vi "Start.vi"(8 "error in (no error)":errorcluster, 10 "Message in":refnum<class "StartMessage.lvclass">, 11 "BMC in":refnum<class "BMC.lvclass">) -> (0 "error out":errorcluster, 3 "BMC out":refnum<class "BMC.lvclass">)   [LabVIEW 2012, in "BMC.lvclass"]
doc: "This member function is called when the statemachine in the run.vi receives an 'start' command. It relays the message to all observers of the component.\n\nOverride this member function in your derived class if you need additional start functionality (but don't forget to call the parent method)."
uses:
  BMC.lvclass
  <vilib>/Distrio/Murmex/StartMessage/StartMessage.lvclass
  <vilib>/Distrio/Murmex/Murmex/Murmex.lvclass
  BMC.lvclass/BMC.ctl
panel:
  # "This member function is called when the statemachine in the run.vi receives an 'start' command. It relays the message to all observers of the component.\n\nOverride this member function in your derived class if you need additional start functionality (but don't forget to call the parent method)."
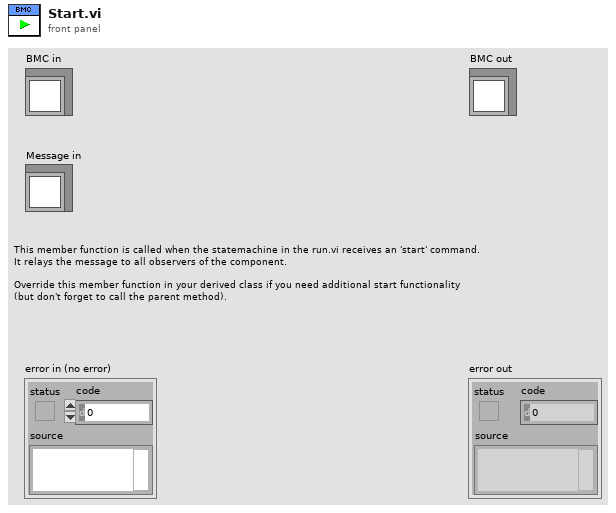
[diagram p1: front panel]
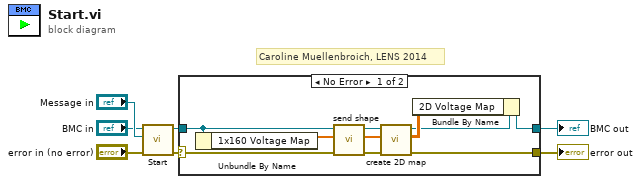
[diagram p0: block diagram]
diagram:
  # "Caroline Muellenbroich, LENS 2014"
  n1 = call-parent "Start.vi"("error in (no error)"="error in (no error)", "Message in"="Message in", "Murmex in"="BMC in") -> ("error out"=w4:errorcluster, "Murmex out"=w2:refnum<class "BMC.lvclass">)  [unwired: 7 in]
  n2 = case shown="No Error" w4 {
    selector: w4 -> [w16 w17]
    tunnel: [w12 w17] -> w3
    tunnel: [w8 w18] -> w1
    tunnel: w2 -> [w15 w18]
    frame No Error {
      n3 = Unbundle By Name(w15) -> ("1x160 Voltage Map"=w14:dbl[])
      n4 = call-dynamic "send shape.vi"("error in (no error)"=w16, "1x160 Voltage Map"=w14, "BMC in"=w15) -> ("error out"=w13:errorcluster, "BMC out"=w11:refnum<class "BMC.lvclass">)  [unwired: 7 in]
      n5 = call-dynamic "create 2D map.vi"("error in (no error)"=w13, "Voltage array"=w14, "BMC in"=w11) -> ("error out"=w12:errorcluster, "2D Voltage Map"=w10:dbl[][], "BMC out"=w9:refnum<class "BMC.lvclass">)  [unwired: 6 in]
      n6 = Bundle By Name(cluster=w9, "2D Voltage Map"=w10) -> (w8:refnum<class "BMC.lvclass">)
    }
    frame Error {
    }
  }
  "error out" <- w3
  "BMC out" <- w1
